vi "cdaq_dds_test.vi"() -> ()   [LabVIEW 2020]
uses:
  <vilib>/DAQmx/write.llb/DAQmx Write (Analog 1D DBL 1Chan NSamp).vi
  <vilib>/DAQmx/create/channels.llb/DAQmx Create Channel (AO-Voltage-Basic).vi
  <vilib>/DAQmx/configure/timing.llb/DAQmx Timing (Sample Clock).vi
  <vilib>/DAQmx/miscellaneous.llb/DAQmx Fill In Error Info.vi
  <resource>/objmgr/daqmx.rc
panel:
  out "wt":dbl
  out "error out":errorcluster
  in  "stop":bool
  in  "rate [Sa/s]":dbl=1000.0 format="%#_13g"
  in  "A [V]":dbl
  in  "f [Hz]":dbl
  in  "DAC device":tag="cDAQ3Mod7"
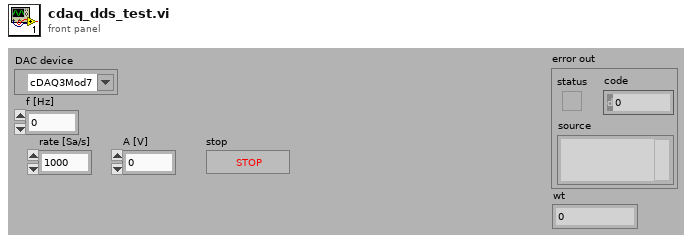
[diagram p1: front panel]
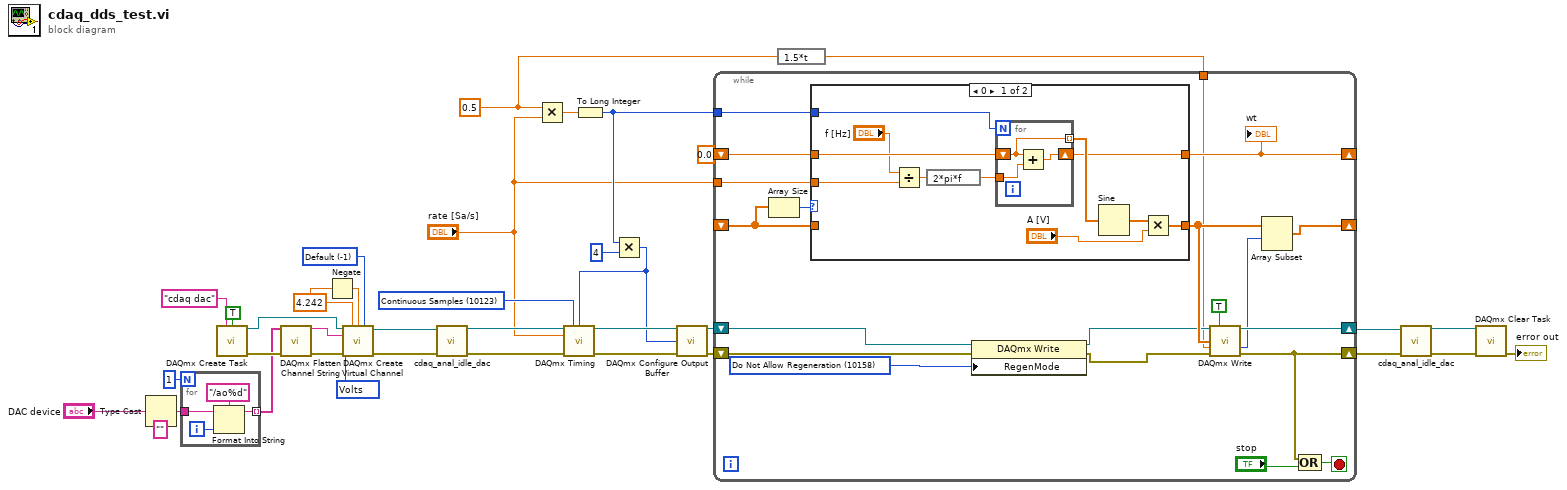
[diagram p0: block diagram]
diagram:
  w8 = 0.5
  w18 = 10123 items=["Finite Samples"=10178, "Continuous Samples"=10123, "Hardware Timed Single Point"=12522] ("sample mode")
  w24 = 4.242 ("maximum value")
  w26 = -1 items=["Default"=-1, "RSE"=10083, "Differential"=10106, "Pseudodifferential"=12529] ("output terminal configuration")
  w31 = 10348 items=["Volts"=10348, "From Custom Scale"=10065] ("units")
  n1 = Type Cast(type="", x="DAC device") -> (*(type *) &x=w29:string)
  n2 = for {
    N: 1 -> [_]
    tunnel: w29 -> [w40]
    tunnel: [w38] -> w33 mode=indexing
    i -> [w39]
    n3 = Format Into String(format string="/ao%d", initial string=w40, w39) -> (resulting string=w38:string)  [unwired: 1 in, 1 out]
  }
  n4 = call <vilib>:"DAQmx Create Task.vi"("new task name"="cdaq dac", "auto cleanup"=TRUE) -> ("task out"=w36:refnum<k21>, "error out"=w35:errorcluster)  [unwired: 12 in]
  n5 = call <vilib>:"DAQmx Flatten Channel String.vi"("names in"=w33, "error in"=w35) -> ("names out"=w32:string, "error out"=w34:errorcluster)  [unwired: 12 in]
  n6 = Negate(x=w24) -> (-x=w25:dbl)
  n7 = call-poly <vilib>:"DAQmx Create Virtual Channel.vi"("task in"=w36, "maximum value"=w24, "minimum value"=w25, "output terminal configuration"=w26, "physical channels"=w32, "units"=w31, "error in"=w34) -> ("task out"=w21:refnum<k21>, "error out"=w22:errorcluster)  [unwired: 7 in]
  n8 = call "cdaq_anal_idle_dac.vi"("error in"=w22, "task in"=w21) -> ("error out"=w20:errorcluster, "task out"=w19:refnum<k21>)  [unwired: 8 in]
  n9 = Multiply(x=w8, y="rate [Sa/s]") -> (x*y=w11:dbl)
  n10 = To Long Integer(number=w11) -> (32bit integer=w10:i32)
  n11 = Multiply(x=w10, y=4) -> (x*y=w2:i32)
  n12 = call-poly <vilib>:"DAQmx Timing.vi"("task/channels in"=w19, "sample mode"=w18, "samples per channel"=w2, "rate"="rate [Sa/s]", "error in"=w20) -> ("task out"=w3:refnum<k21>, "error out"=w6:errorcluster)  [unwired: 9 in]
  n13 = call <vilib>:"DAQmx Configure Output Buffer.vi"("task/channels in"=w3, "buffer size (in samples per channel)"=w2, "error in"=w6) -> ("task out"=w4:refnum<k21>, "error out"=w5:errorcluster)  [unwired: 11 in]
  n14 = expression code="1.5*t"(w8) -> (w7:dbl)
  n15 = while {
    shift-right: [w51] -> w16
    shift-left: w5 -> [w48]
    shift-right: [w60] -> w15
    shift-left: w4 -> [w49]
    shift-right: [w58] -> _
    shift-left: 0.0 -> [w59]
    shift-right: [w56] -> _
    shift-left: _ -> [w53]
    tunnel: w10 -> [w45]
    tunnel: w7 -> [w44]
    tunnel: "rate [Sa/s]" -> [w42]
    stop <- w52 stop-if-true
    w43 = 10158 items=["Allow Regeneration"=10097, "Do Not Allow Regeneration"=10158] ("RegenMode")
    n16 = Array Size(array=w53) -> (size(s)=w54:i32)
    n17 = case shown="0" w54 {
      tunnel: w59 -> [w72 w77]
      tunnel: [w68 w76] -> w57
      tunnel: [w69 w77] -> w58
      tunnel: w53 -> [_ w76]
      tunnel: w45 -> [w66 _]
      tunnel: w42 -> [w63 _]
      frame 0 {
        n18 = Divide(x="f [Hz]", y=w63) -> (x/y=w64:dbl)
        n19 = expression code="2*pi*f"(w64) -> (w65:dbl)
        n20 = for {
          N: w66 -> [_]
          shift-right: [w75] -> w69
          shift-left: w72 -> [w73]
          tunnel: w65 -> [w74]
          tunnel: [w73] -> w71 mode=indexing
          n21 = Add(x=w73, y=w74) -> (x+y=w75:dbl)
        }
        n22 = Sine(x=w71) -> (sin(x)=w70:dbl[])
        n23 = Multiply(x=w70, y="A [V]") -> (x*y=w68:dbl[])
      }
      frame Default {
      }
    }
    "wt" <- w58
    n24 = property class="DAQmx Write"(reference=w49, error in=w48, "RegenMode"=w43) -> (reference out=w47:refnum<k21>, error out=w46:errorcluster)
    n25 = call-poly <vilib>:"DAQmx Write.vi"("task/channels in"=w47, "auto start"=TRUE, "data"=w57, "timeout"=w44, "error in"=w46) -> ("task out"=w60:refnum<k21>, "number of samples written per channel"=w55:u32, "error out"=w51:errorcluster)  [unwired: 8 in]
    n26 = Array Subset(array=w57, index=w55) -> (w56:dbl[])  [unwired: 1 in]
    n27 = Compound Arithmetic op=OR(w51, "stop") -> (w52:bool)
  }
  n28 = call "cdaq_anal_idle_dac.vi"("error in"=w16, "task in"=w15) -> ("error out"=w14:errorcluster, "task out"=w13:refnum<k21>)  [unwired: 8 in]
  n29 = call <vilib>:"DAQmx Clear Task.vi"("task in"=w13, "error in"=w14) -> ("error out"=→"error out":errorcluster)  [unwired: 13 in]
